vi "PSAE_VCH_VCH List.vi"(8 "Error In (no error)":errorcluster) -> (0 "Error Out":errorcluster, 3 "VCHList":T1)   [LabVIEW 2016]
uses:
  VCH/Private/Ctrls/PSVCH_All Channels.ctl
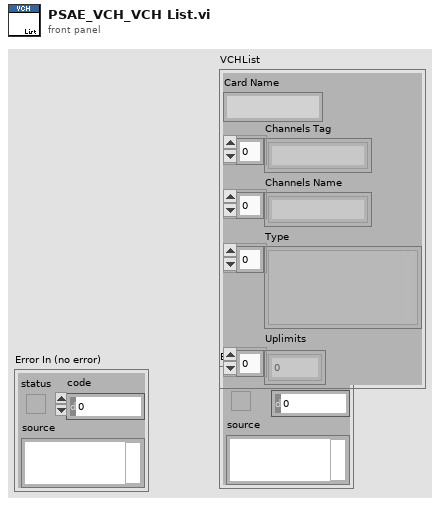
[diagram p1: front panel]
types:
  T1 = typedef "PSVCH_All Channels.ctl" = cluster{"Card Name":string, "Channels Tag":string[], "Channels Name":string[], "Type":variant[], "Uplimits":dbl[]}
  T2 = typedef "PSVCH_VCH Info.ctl" = cluster{"Tag":string[], "Tag String":string[], "Name":string[], "Enable":bool[], "Formula":string[], "Unit":string[], "Save":bool[], "Time":i64[]}
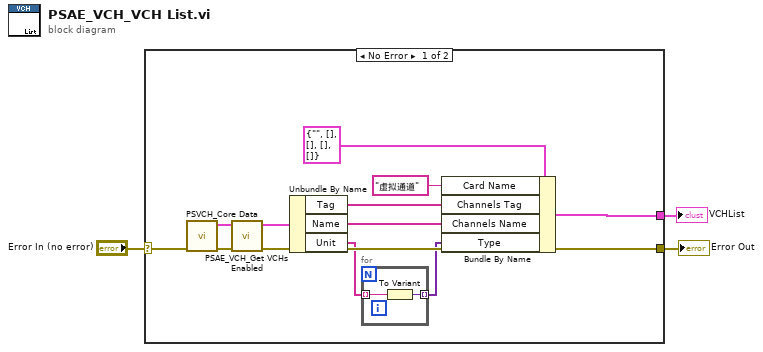
[diagram p0: block diagram]
diagram:
  n1 = case shown="No Error" "Error In (no error)" {
    selector: "Error In (no error)" -> [w15 w18]
    tunnel: [w7 w18] -> w2
    tunnel: [w6 _] -> w1
    frame No Error {
      n2 = call "PSVCH_Core Data.vi"("Error In (no error)"=w15) -> ("Error Out"=w14:errorcluster, "VCH Out"=w13:T2)  [unwired: 9 in]
      n3 = call "PSAE_VCH_Get VCHs Enabled.vi"("Error In"=w14, "VCH"=w13) -> ("Error Out"=w7:errorcluster, "VCH"=w12:T2)  [unwired: 8 in]
      n4 = Unbundle By Name(w12) -> ("Tag"=w9:string[], "Name"=w8:string[], "Unit"=w5:string[])
      n5 = for {
        tunnel: w5 -> [w17] mode=indexing
        tunnel: [w16] -> w4 mode=indexing
        n6 = To Variant(anything=w17) -> (Variant=w16:variant)
      }
      n7 = Bundle By Name(cluster=T1 {"Card Name"="", "Channels Tag"=[], "Channels Name"=[], "Type"=[], "Uplimits"=[]} ("DAQ2ANA"), "Card Name"="虚拟通道", "Channels Tag"=w9, "Channels Name"=w8, "Type"=w4) -> (w6:T1)
    }
    frame Error {
    }
  }
  "Error Out" <- w2
  "VCHList" <- w1
